vi "Get_All_detections_JSON.vi"(2 "path":path) -> (5 "annotated_image":string, 6 "detection":T1(array[cluster]))   [LabVIEW 2024]
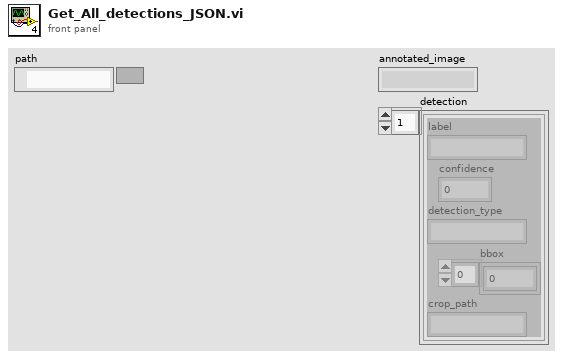
[diagram p1: front panel]
types:
  T1 = cluster{"label":string, "confidence":i32, "detection_type":string, "bbox":dbl[], "crop_path":string}[]
  T2 = cluster{"annotated_image":string, "detections":cluster{"label":string, "confidence":i32, "detection_type":string, "bbox":dbl[], "crop_path":string}[]}
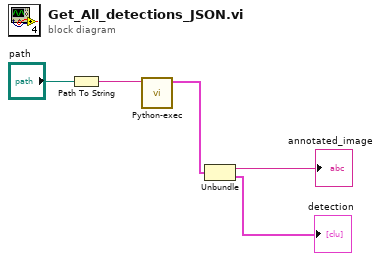
[diagram p0: block diagram]
diagram:
  n1 = Path To String(path="path") -> (string=w4:string)
  n2 = call "Python-exec.vi"("String"=w4) -> ("value"=w3:T2)  [unwired: 10 in]
  n3 = Unbundle(w3) -> ("annotated_image"=→"annotated_image":string, "detections"=→"detection":T1)
